vi "FIFORawDataScreener.vi"(2 "File Type":T2(ring)=enum."48 bit", 3 "Path":path) -> ()   [LabVIEW 2009]
uses:
  <vilib>/Analysis/NI_AALPro.lvlib
  <vilib>/Analysis/NI_AALBase.lvlib
panel:
  out "XY Graph":T1(graph)
  out "Waveform Graph":u32[](graph)
  out "MTOV B&H":dbl
  out "INV B&H":dbl
  out "MTOV & INV B&H":dbl
  out "MTOV & INV LV":dbl
  out "INV LV":dbl
  out "MTOV LV":dbl
  out "Waveform Graph 2":i32[](graph)
  in  "Bin":bool
  in  "proof":bool
  in  "Start":bool
  out "RawData":string[][](table)
  in  "Exit":bool
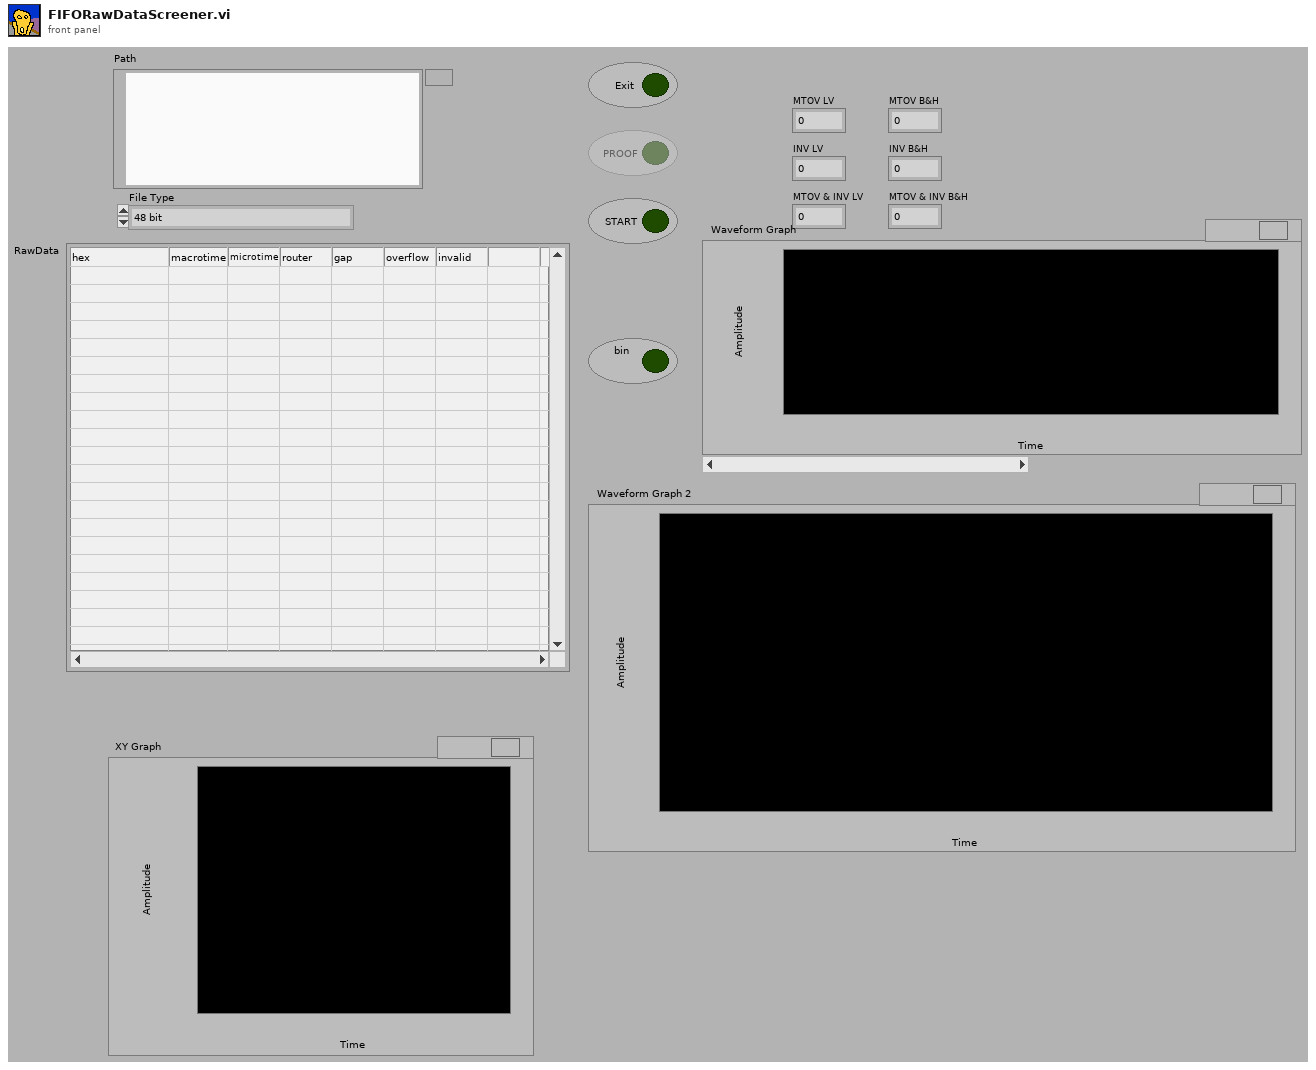
[diagram p1: front panel]
types:
  T1 = cluster{"X Values":dbl[], "Histogram: h(x)":i32[]}
  T2 = enum16{"32 bit", "48 bit", "48 bit (swapped bytes)", "32bit SPC830/130 LV Style", "32bit SPC830/130 B&H Style"}
  T3 = cluster{"router channels":u8[], "macro times":u32[], "micro times":u16[], "invalid times":u32[], "gap times":u32[]}
  T4 = enum16{"open", "open or create", "create or replace", "create", "open (read only)"}
  T5 = enum16{"Left Button", "Center Button", "Right Button", "Window Close"}
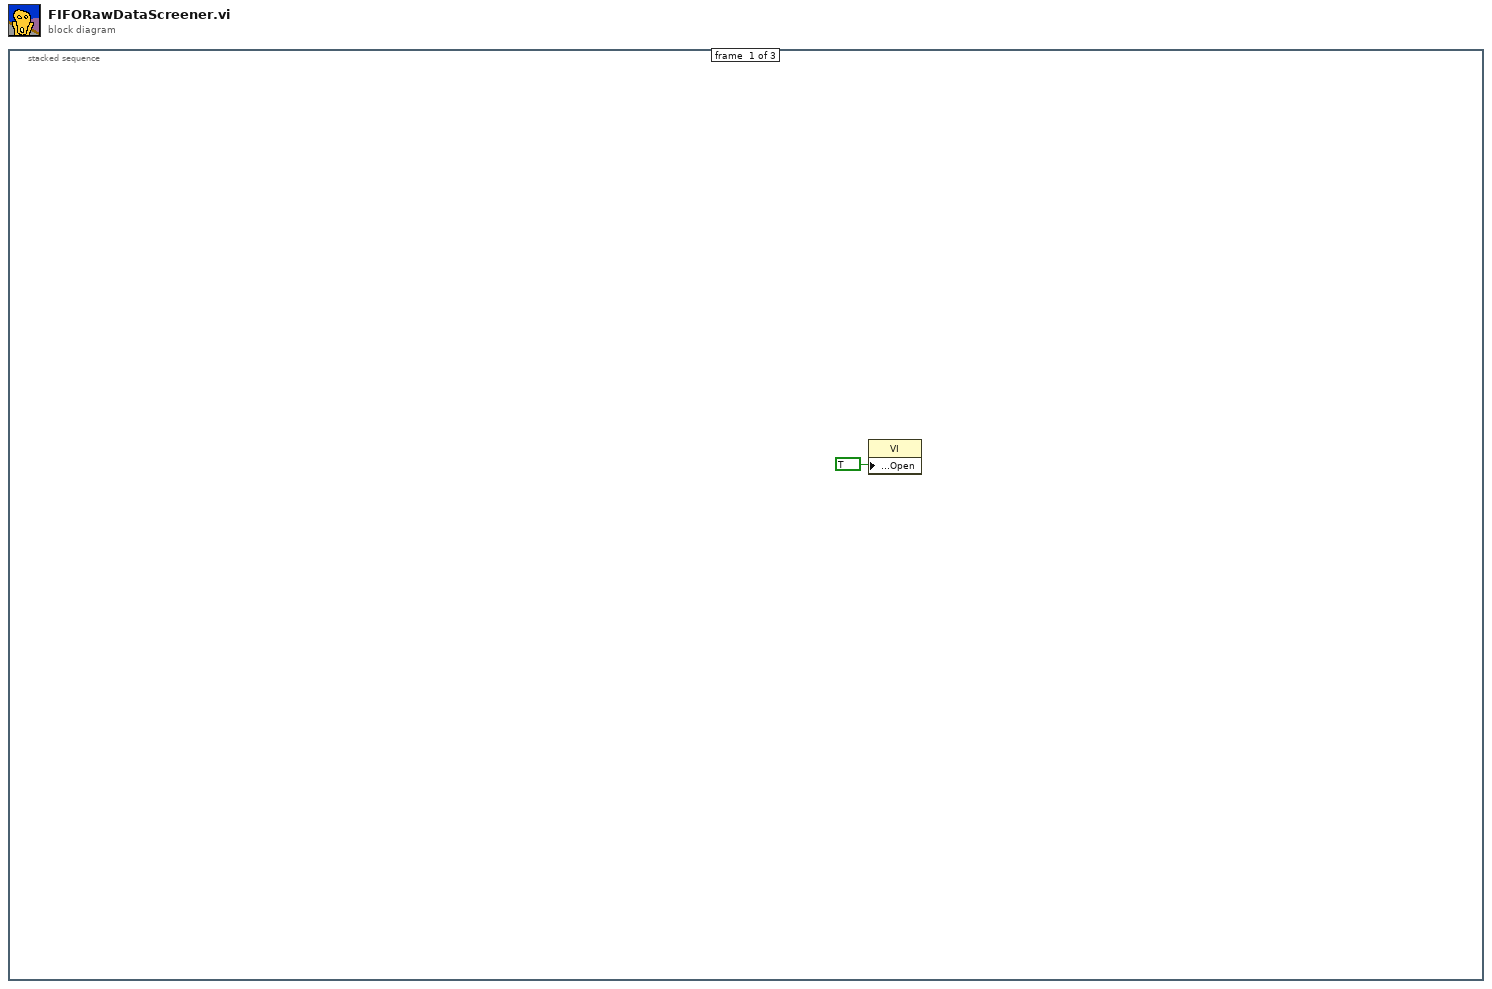
[diagram p0: block diagram]
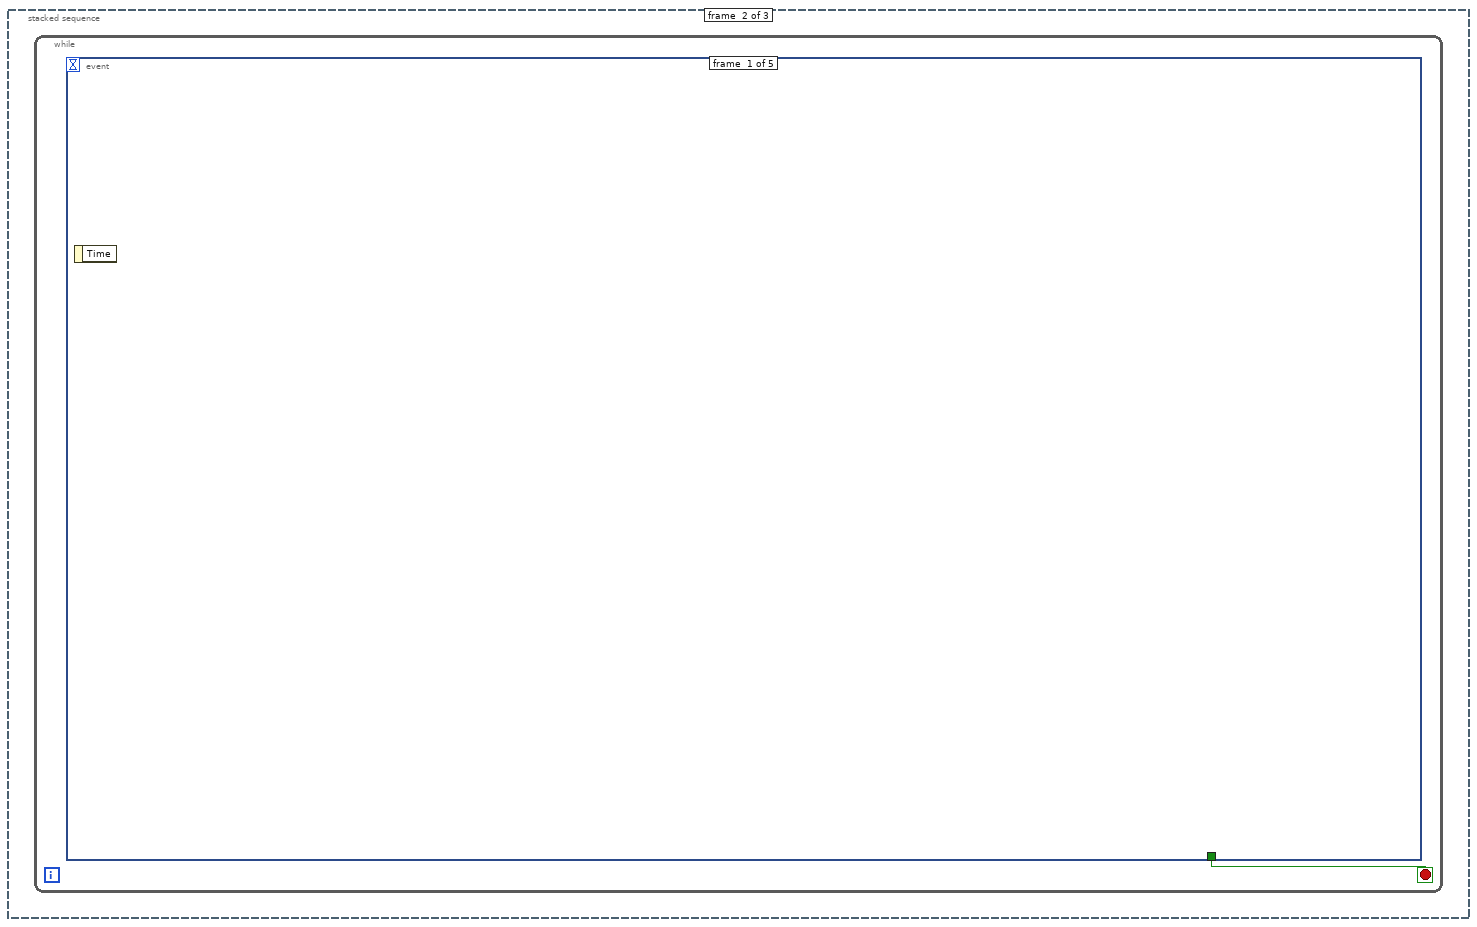
[diagram p2: hidden frame]
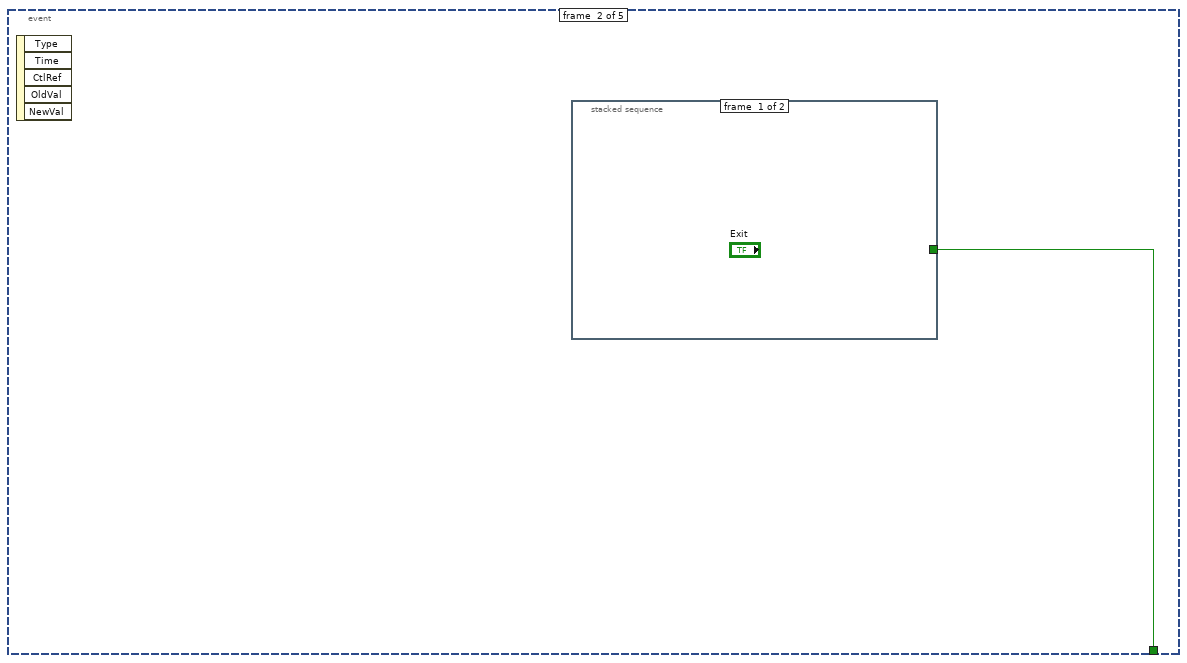
[diagram p3: hidden frame]
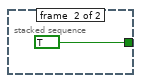
[diagram p4: hidden frame]
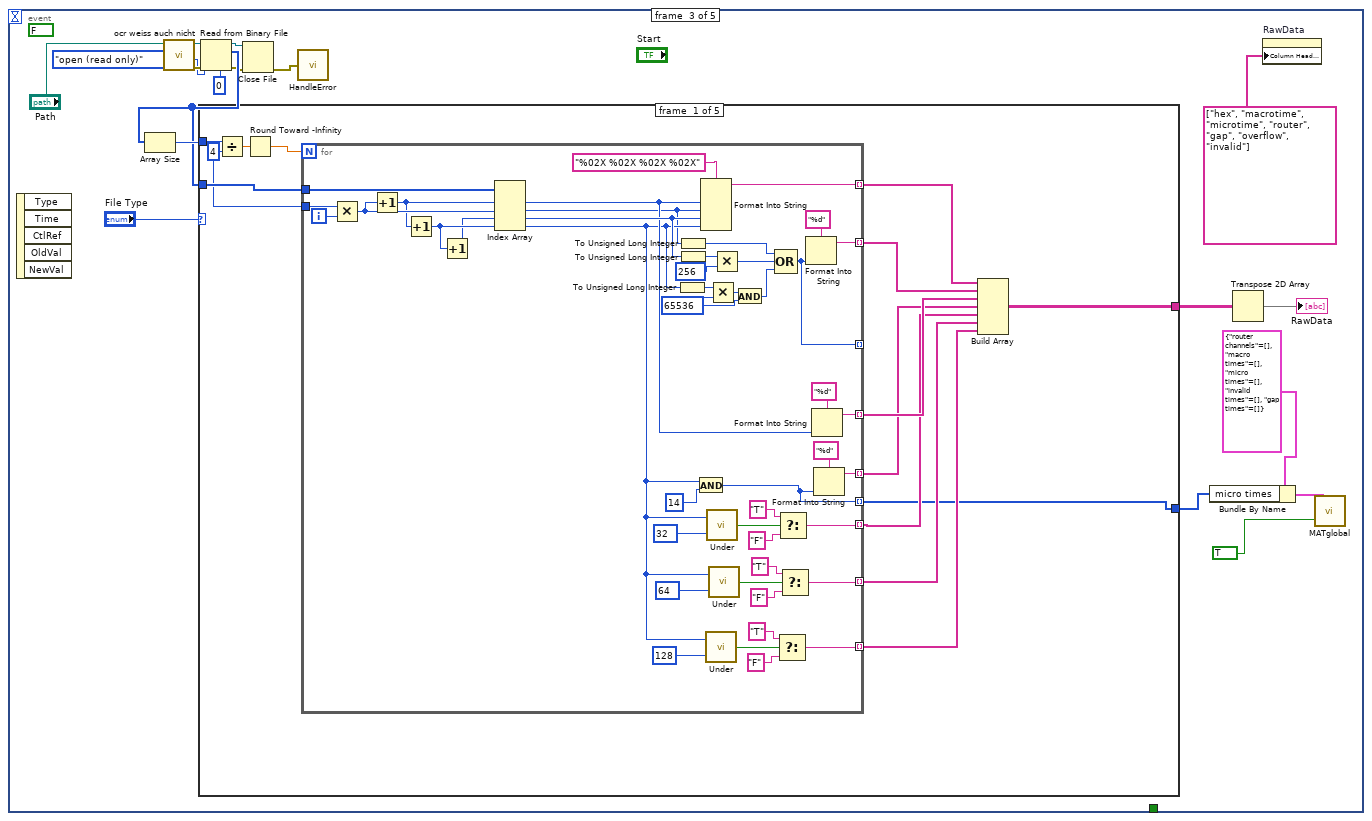
[diagram p5: hidden frame]
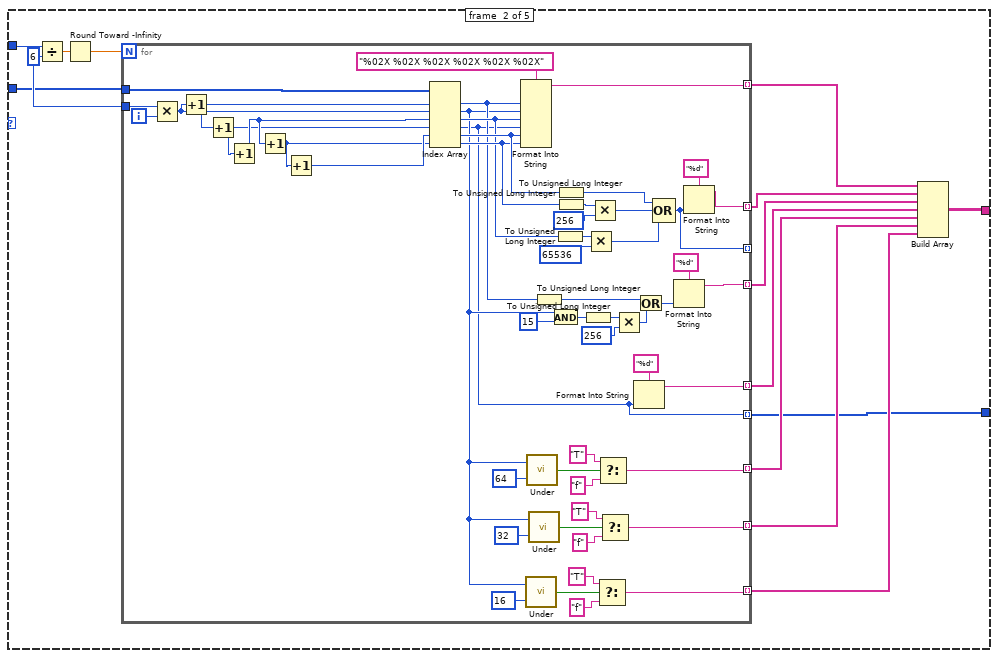
[diagram p6: hidden frame]
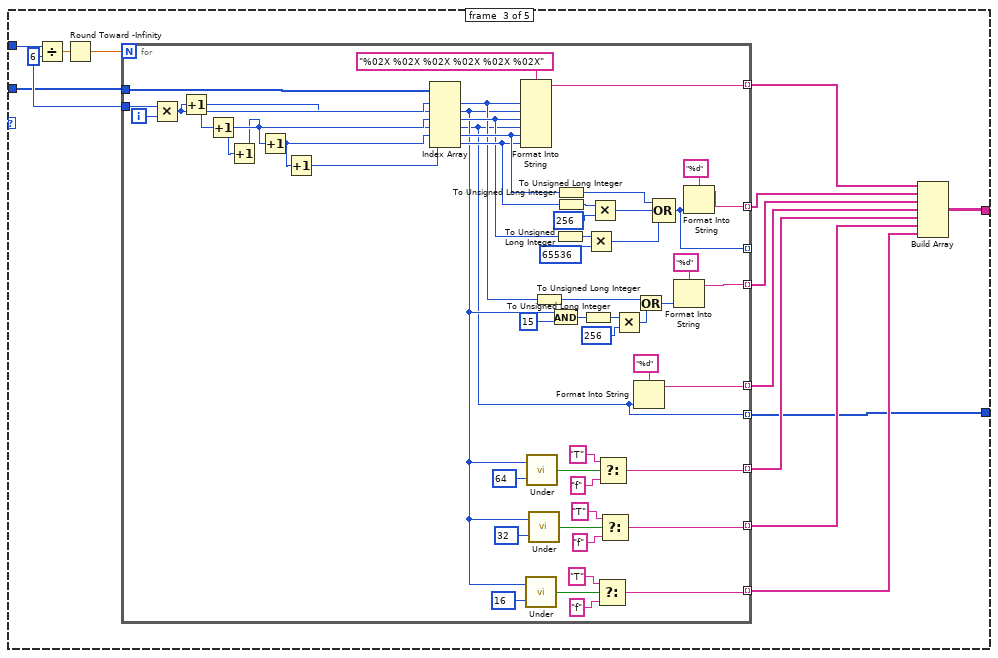
[diagram p7: hidden frame]
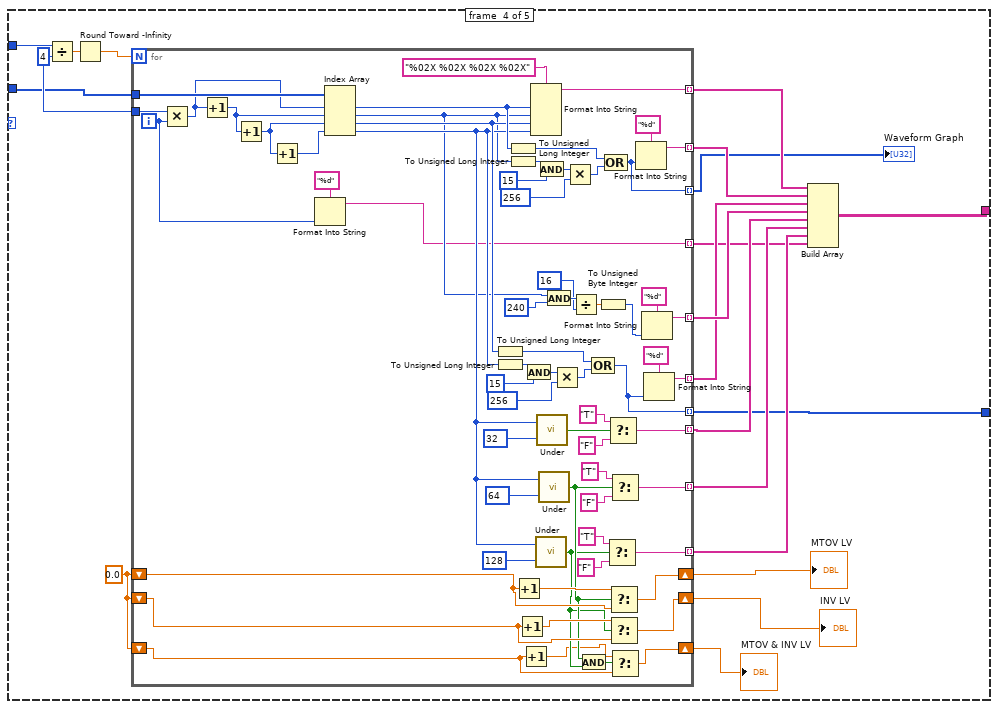
[diagram p8: hidden frame]
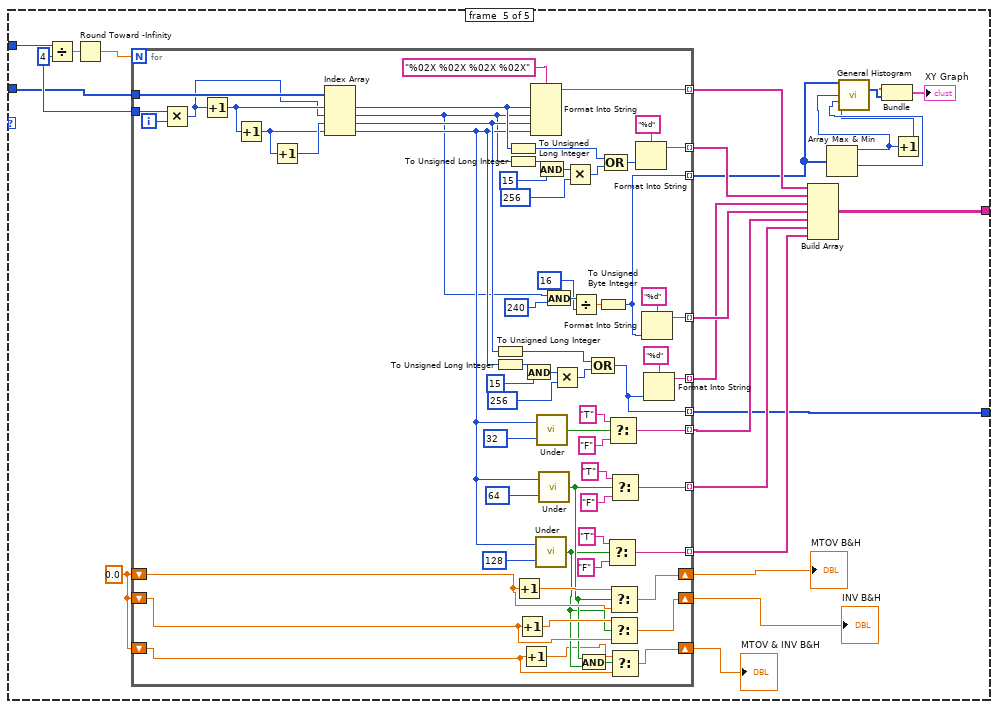
[diagram p9: hidden frame]
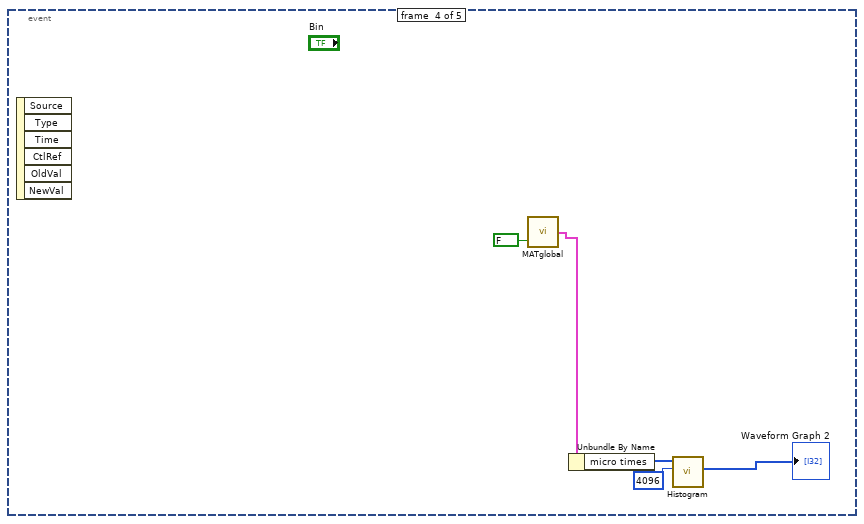
[diagram p10: hidden frame]
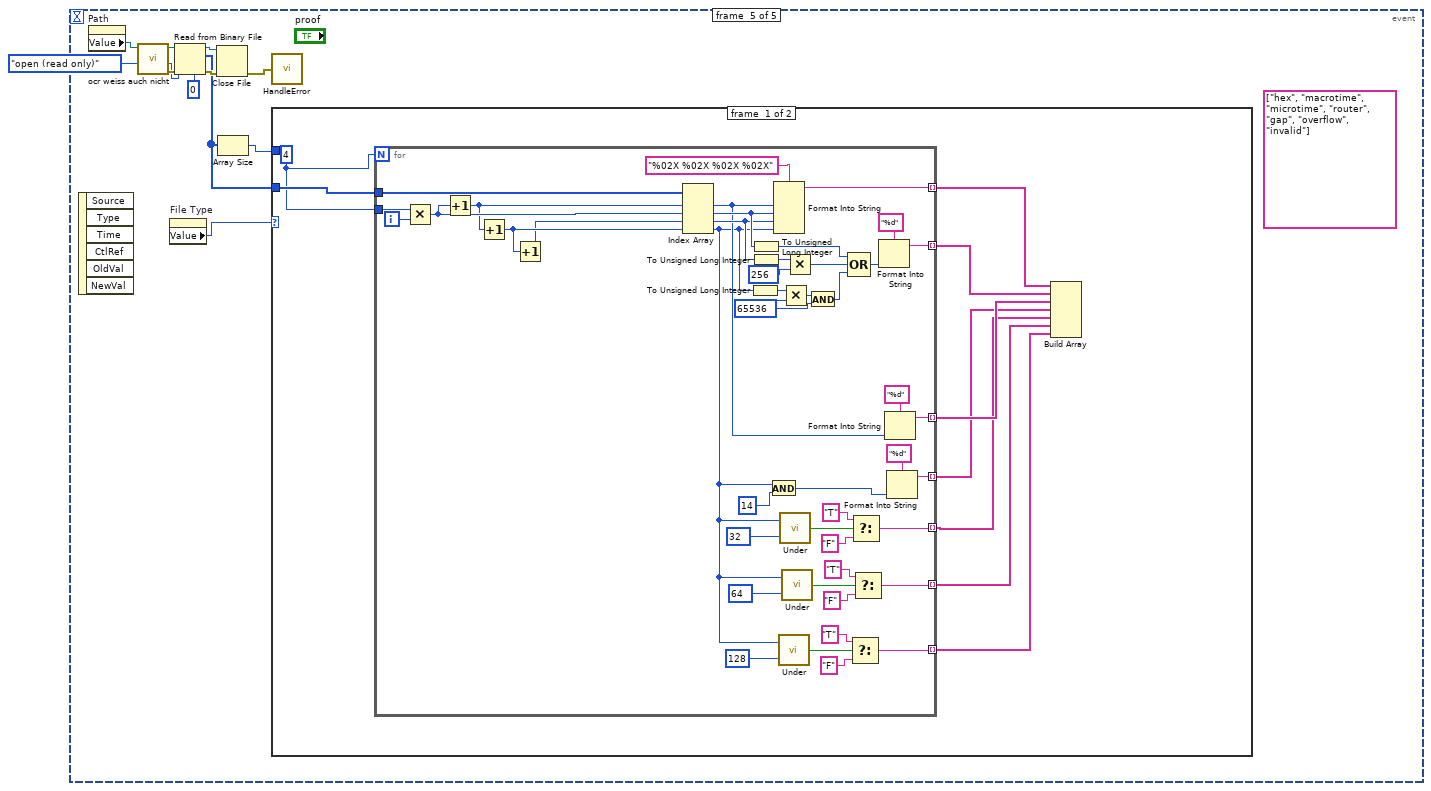
[diagram p11: hidden frame]
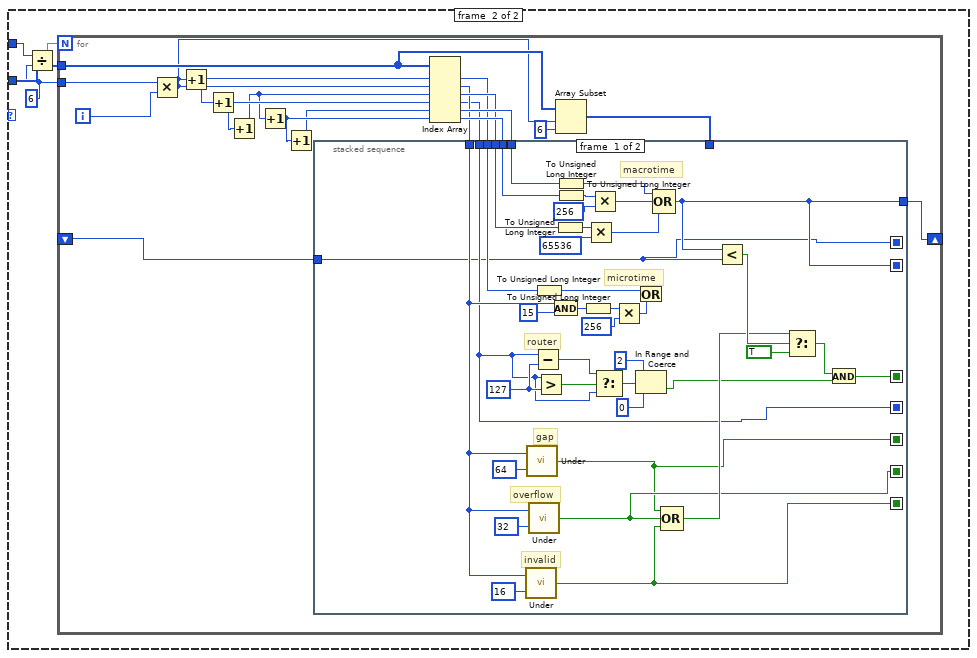
[diagram p12: hidden frame]
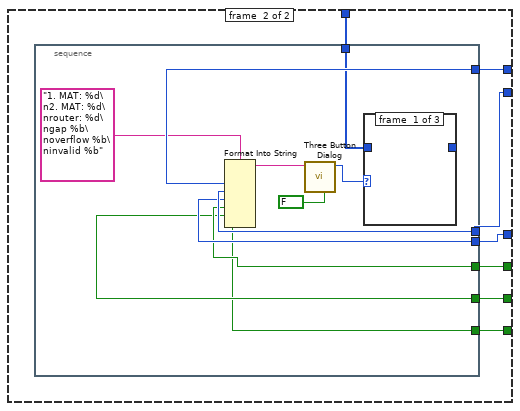
[diagram p14: hidden frame]
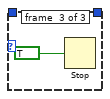
[diagram p16: hidden frame]
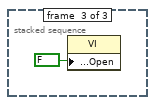
[diagram p17: hidden frame]
diagram:
  n1 = stacked-sequence {
    frame #0 {
      n2 = property class="VI"("Front Panel Window:Open"=TRUE) -> ()  [unwired: 2 in, 2 out]
    }
    frame #1 {
      n3 = while {
        stop <- w2 stop-if-true
        n4 = event shown="[2] \"Path\", \"File Type\", \"Start\": Value Change" {
          selector: _ -> [_ _ _ _ _]
          dyn-events: _ -> [_ _ _ _ _]
          timeout: _ -> [_ _ _ _ _]
          tunnel: [_ w3 _ _ _] -> w2
          event #0 {
            n5 = event-data() -> ()  [unwired: 1 in, 1 out]
          }
          event #1 {
            n6 = event-data() -> ()  [unwired: 1 in, 5 out]
            n7 = stacked-sequence {
              tunnel: [_ TRUE] -> w3
              frame #0 {
              }
              frame #1 {
              }
            }
          }
          event #2 {
            (unwired) FALSE
            n8 = event-data() -> ()  [unwired: 1 in, 5 out]
            n9 = call "ocr weiss auch nicht.vi"("function (open:0)"=T4."open (read only)", "file path"="Path") -> ("error out"=w15:errorcluster, "file size (bytes)"=w11:i32, "refnum"=w16:refnum<file>)  [unwired: 6 in, 1 out]
            n10 = Read from Binary File(5:u8 0 ("byte stream type"), 8:w15, 10:w11, 11:w16) -> (0:w12:errorcluster, 2:w21:u8[], 3:w13:refnum<file>)  [unwired: 2 in, 1 out]
            n11 = Array Size(array=w21) -> (size(s)=w22:i32)
            n12 = case shown="\"32bit SPC830/130 B&H Style\"" "File Type" {
              tunnel: w22 -> [w37 w86 w153 w227 w317]
              tunnel: w21 -> [w35 w83 w150 w228 w318]
              tunnel: [w25 w85 w152 w226 w316] -> w20
              tunnel: [w24 w84 w151 w223 w313] -> w5
              frame #0 {
                w34 = 4 ("y")
                n13 = Divide(x=w37, y=w34) -> (x/y=w36:dbl)
                n14 = Round Toward -Infinity(1:w36) -> (0:w33:dbl)
                n15 = for {
                  N: w33 -> [_]
                  tunnel: w35 -> [w82]
                  tunnel: w34 -> [w80]
                  tunnel: [w79] -> w32 mode=indexing
                  tunnel: [w68] -> w31 mode=indexing
                  tunnel: [w65] -> w30 mode=indexing
                  tunnel: [w63] -> w29 mode=indexing
                  tunnel: [w58] -> w28 mode=indexing
                  tunnel: [w49] -> w27 mode=indexing
                  tunnel: [w48] -> w26 mode=indexing
                  tunnel: [w39] -> _ mode=indexing
                  tunnel: [w38] -> w24 mode=indexing
                  i -> [w81]
                  w73 = u32 65536 ("y")
                  n16 = Multiply(x=w80, y=w81) -> (x*y=w44:i32)
                  n17 = Increment(x=w44) -> (x+1=w43:i32)
                  n18 = Increment(x=w43) -> (x+1=w42:i32)
                  n19 = Increment(x=w42) -> (x+1=w41:i32)
                  n20 = Index Array(array=w82, index #1=w43, index #2=w44, index #3=w41, index #4=w42) -> (element #1=w66:u8, element #2=w40:u8, element #3=w78:u8, element #4=w46:u8)
                  n21 = To Unsigned Long Integer(number=w46) -> (unsigned 32bit integer=w75:u32)
                  n22 = To Unsigned Long Integer(number=w40) -> (unsigned 32bit integer=w72:u32)
                  n23 = To Unsigned Long Integer(number=w78) -> (unsigned 32bit integer=w77:u32)
                  n24 = And(x=w46, y=u8 14) -> (x .and. y?=w38:u8)
                  n25 = Format Into String(format string="%02X %02X %02X %02X", w66, w40, w78, w46) -> (resulting string=w79:string)  [unwired: 2 in, 1 out]
                  n26 = call "Under.vi"("y"=u8 128, "byte stream type"=w46) -> ("Boolean"=w52:bool)
                  n27 = call "Under.vi"("y"=u8 32, "byte stream type"=w46) -> ("Boolean"=w61:bool)
                  n28 = Multiply(x=w75, y=w73) -> (x*y=w74:u32)
                  n29 = call "Under.vi"("y"=u8 64, "byte stream type"=w46) -> ("Boolean"=w55:bool)
                  n30 = Multiply(x=w77, y=u32 256) -> (x*y=w71:u32)
                  n31 = And(x=w74, y=w73) -> (x .and. y?=w70:u32)
                  n32 = Compound Arithmetic op=OR(w72, w71, w70) -> (w39:u32)
                  n33 = Select(t="T" ("format string"), s=w52, f="F" ("format string")) -> (s? t:f=w48:string)
                  n34 = Select(t="T" ("format string"), s=w61, f="F" ("format string")) -> (s? t:f=w58:string)
                  n35 = Select(t="T" ("format string"), s=w55, f="F" ("format string")) -> (s? t:f=w49:string)
                  n36 = Format Into String(format string="%d", w39) -> (resulting string=w68:string)  [unwired: 2 in, 1 out]
                  n37 = Format Into String(format string="%d", w66) -> (resulting string=w65:string)  [unwired: 2 in, 1 out]
                  n38 = Format Into String(format string="%d", w38) -> (resulting string=w63:string)  [unwired: 2 in, 1 out]
                }
                n39 = Build Array(w32, w31, w30, w29, w28, w27, w26) -> (w25:string[][])
              }
              frame #1 {
                w88 = 6 ("y")
                n40 = Divide(x=w86, y=w88) -> (x/y=w87:dbl)
                n41 = Round Toward -Infinity(1:w87) -> (0:w89:dbl)
                n42 = for {
                  N: w89 -> [_]
                  tunnel: w83 -> [w149]
                  tunnel: w88 -> [w147]
                  tunnel: [w145] -> w90 mode=indexing
                  tunnel: [w138] -> w91 mode=indexing
                  tunnel: [w136] -> w92 mode=indexing
                  tunnel: [w134] -> w93 mode=indexing
                  tunnel: [w129] -> w94 mode=indexing
                  tunnel: [w120] -> w95 mode=indexing
                  tunnel: [w119] -> w96 mode=indexing
                  tunnel: [w104] -> _ mode=indexing
                  tunnel: [w103] -> w84 mode=indexing
                  i -> [w148]
                  n43 = Multiply(x=w147, y=w148) -> (x*y=w101:i32)
                  n44 = Increment(x=w101) -> (x+1=w102:i32)
                  n45 = Increment(x=w102) -> (x+1=w99:i32)
                  n46 = Increment(x=w99) -> (x+1=w100:i32)
                  n47 = Increment(x=w100) -> (x+1=w97:i32)
                  n48 = Increment(x=w97) -> (x+1=w98:i32)
                  n49 = Index Array(array=w149, index #1=w102, index #2=w101, index #3=w100, index #4=w99, index #5=w98, index #6=w97) -> (element #1=w114:u8, element #2=w105:u8, element #3=w115:u8, element #4=w103:u8, element #5=w117:u8, element #6=w116:u8)
                  n50 = Format Into String(format string="%02X %02X %02X %02X %02X %02X", w114, w105, w115, w103, w117, w116) -> (resulting string=w145:string)  [unwired: 2 in, 1 out]
                  n51 = call "Under.vi"("y"=u8 16, "byte stream type"=w105) -> ("Boolean"=w123:bool)
                  n52 = call "Under.vi"("y"=u8 64, "byte stream type"=w105) -> ("Boolean"=w132:bool)
                  n53 = call "Under.vi"("y"=u8 32, "byte stream type"=w105) -> ("Boolean"=w126:bool)
                  n54 = To Unsigned Long Integer(number=w114) -> (unsigned 32bit integer=w109:u32)
                  n55 = And(x=w105, y=u8 15) -> (x .and. y?=w107:u8)
                  n56 = To Unsigned Long Integer(number=w115) -> (unsigned 32bit integer=w142:u32)
                  n57 = To Unsigned Long Integer(number=w117) -> (unsigned 32bit integer=w141:u32)
                  n58 = To Unsigned Long Integer(number=w116) -> (unsigned 32bit integer=w144:u32)
                  n59 = To Unsigned Long Integer(number=w107) -> (unsigned 32bit integer=w111:u32)
                  n60 = Multiply(x=w142, y=u32 65536) -> (x*y=w110:u32)
                  n61 = Multiply(x=w144, y=u32 256) -> (x*y=w140:u32)
                  n62 = Select(t="T" ("format string"), s=w123, f="f" ("format string")) -> (s? t:f=w119:string)
                  n63 = Select(t="T" ("format string"), s=w132, f="f" ("format string")) -> (s? t:f=w129:string)
                  n64 = Select(t="T" ("format string"), s=w126, f="f" ("format string")) -> (s? t:f=w120:string)
                  n65 = Multiply(x=w111, y=u32 256) -> (x*y=w108:u32)
                  n66 = Format Into String(format string="%d", w103) -> (resulting string=w134:string)  [unwired: 2 in, 1 out]
                  n67 = Or(x=w109, y=w108) -> (x .or. y?=w113:u32)
                  n68 = Compound Arithmetic op=OR(w141, w140, w110) -> (w104:u32)
                  n69 = Format Into String(format string="%d", w113) -> (resulting string=w136:string)  [unwired: 2 in, 1 out]
                  n70 = Format Into String(format string="%d", w104) -> (resulting string=w138:string)  [unwired: 2 in, 1 out]
                }
                n71 = Build Array(w90, w91, w92, w93, w94, w95, w96) -> (w85:string[][])
              }
              frame #2 {
                w155 = 6 ("y")
                n72 = Divide(x=w153, y=w155) -> (x/y=w154:dbl)
                n73 = Round Toward -Infinity(1:w154) -> (0:w156:dbl)
                n74 = for {
                  N: w156 -> [_]
                  tunnel: w150 -> [w216]
                  tunnel: w155 -> [w214]
                  tunnel: [w212] -> w157 mode=indexing
                  tunnel: [w205] -> w158 mode=indexing
                  tunnel: [w203] -> w159 mode=indexing
                  tunnel: [w201] -> w160 mode=indexing
                  tunnel: [w196] -> w161 mode=indexing
                  tunnel: [w187] -> w162 mode=indexing
                  tunnel: [w186] -> w163 mode=indexing
                  tunnel: [w171] -> _ mode=indexing
                  tunnel: [w170] -> w151 mode=indexing
                  i -> [w215]
                  n75 = Multiply(x=w214, y=w215) -> (x*y=w169:i32)
                  n76 = Increment(x=w169) -> (x+1=w168:i32)
                  n77 = Increment(x=w168) -> (x+1=w167:i32)
                  n78 = Increment(x=w167) -> (x+1=w166:i32)
                  n79 = Increment(x=w166) -> (x+1=w165:i32)
                  n80 = Increment(x=w165) -> (x+1=w164:i32)
                  n81 = Index Array(array=w216, index #1=w169, index #2=w168, index #3=w167, index #4=w166, index #5=w165, index #6=w164) -> (element #1=w181:u8, element #2=w172:u8, element #3=w182:u8, element #4=w170:u8, element #5=w184:u8, element #6=w183:u8)
                  n82 = Format Into String(format string="%02X %02X %02X %02X %02X %02X", w181, w172, w182, w170, w184, w183) -> (resulting string=w212:string)  [unwired: 2 in, 1 out]
                  n83 = call "Under.vi"("y"=u8 16, "byte stream type"=w172) -> ("Boolean"=w190:bool)
                  n84 = call "Under.vi"("y"=u8 64, "byte stream type"=w172) -> ("Boolean"=w199:bool)
                  n85 = call "Under.vi"("y"=u8 32, "byte stream type"=w172) -> ("Boolean"=w193:bool)
                  n86 = To Unsigned Long Integer(number=w181) -> (unsigned 32bit integer=w176:u32)
                  n87 = And(x=w172, y=u8 15) -> (x .and. y?=w174:u8)
                  n88 = To Unsigned Long Integer(number=w182) -> (unsigned 32bit integer=w209:u32)
                  n89 = To Unsigned Long Integer(number=w184) -> (unsigned 32bit integer=w208:u32)
                  n90 = To Unsigned Long Integer(number=w183) -> (unsigned 32bit integer=w211:u32)
                  n91 = To Unsigned Long Integer(number=w174) -> (unsigned 32bit integer=w178:u32)
                  n92 = Multiply(x=w209, y=u32 65536) -> (x*y=w177:u32)
                  n93 = Multiply(x=w211, y=u32 256) -> (x*y=w207:u32)
                  n94 = Select(t="T" ("format string"), s=w190, f="f" ("format string")) -> (s? t:f=w186:string)
                  n95 = Select(t="T" ("format string"), s=w199, f="f" ("format string")) -> (s? t:f=w196:string)
                  n96 = Select(t="T" ("format string"), s=w193, f="f" ("format string")) -> (s? t:f=w187:string)
                  n97 = Multiply(x=w178, y=u32 256) -> (x*y=w175:u32)
                  n98 = Format Into String(format string="%d", w170) -> (resulting string=w201:string)  [unwired: 2 in, 1 out]
                  n99 = Or(x=w176, y=w175) -> (x .or. y?=w180:u32)
                  n100 = Compound Arithmetic op=OR(w208, w207, w177) -> (w171:u32)
                  n101 = Format Into String(format string="%d", w180) -> (resulting string=w203:string)  [unwired: 2 in, 1 out]
                  n102 = Format Into String(format string="%d", w171) -> (resulting string=w205:string)  [unwired: 2 in, 1 out]
                }
                n103 = Build Array(w157, w158, w159, w160, w161, w162, w163) -> (w152:string[][])
              }
              frame #3 {
                w220 = 0.0
                w235 = 4 ("y")
                n104 = Divide(x=w227, y=w235) -> (x/y=w236:dbl)
                n105 = Round Toward -Infinity(1:w236) -> (0:w234:dbl)
                n106 = for {
                  N: w234 -> [_]
                  tunnel: w228 -> [w301]
                  tunnel: w235 -> [w300]
                  tunnel: [w299] -> w233 mode=indexing
                  tunnel: [w296] -> w232 mode=indexing
                  tunnel: [w294] -> w225 mode=indexing
                  tunnel: [w292] -> w224 mode=indexing
                  tunnel: [w287] -> w231 mode=indexing
                  tunnel: [w281] -> w230 mode=indexing
                  tunnel: [w280] -> w229 mode=indexing
                  tunnel: [w241] -> w223 mode=indexing
                  shift-right: [w249] -> w222
                  shift-left: w220 -> [w250]
                  shift-right: [w254] -> w221
                  shift-left: w220 -> [w253]
                  shift-right: [w248] -> w219
                  shift-left: w220 -> [w243]
                  tunnel: [w240] -> w218 mode=indexing
                  tunnel: [w237] -> w217 mode=indexing
                  i -> [w238]
                  n107 = Multiply(x=w300, y=w238) -> (x*y=w259:i32)
                  n108 = Increment(x=w259) -> (x+1=w258:i32)
                  n109 = Increment(x=w258) -> (x+1=w257:i32)
                  n110 = Increment(x=w257) -> (x+1=w256:i32)
                  n111 = Format Into String(format string="%d", w238) -> (resulting string=w237:string)  [unwired: 2 in, 1 out]
                  n112 = Index Array(array=w301, index #1=w259, index #2=w258, index #3=w257, index #4=w256) -> (element #1=w278:u8, element #2=w263:u8, element #3=w266:u8, element #4=w265:u8)
                  n113 = To Unsigned Long Integer(number=w266) -> (unsigned 32bit integer=w267:u32)
                  n114 = To Unsigned Long Integer(number=w265) -> (unsigned 32bit integer=w269:u32)
                  n115 = To Unsigned Long Integer(number=w278) -> (unsigned 32bit integer=w298:u32)
                  n116 = To Unsigned Long Integer(number=w263) -> (unsigned 32bit integer=w276:u32)
                  n117 = Increment(x=w250) -> (x+1=w251:dbl)
                  n118 = Increment(x=w253) -> (x+1=w252:dbl)
                  n119 = Increment(x=w243) -> (x+1=w244:dbl)
                  n120 = And(x=w269, y=u32 15) -> (x .and. y?=w270:u32)
                  n121 = Format Into String(format string="%02X %02X %02X %02X", w278, w263, w266, w265) -> (resulting string=w299:string)  [unwired: 2 in, 1 out]
                  n122 = call "Under.vi"("y"=u8 128, "byte stream type"=w265) -> ("Boolean"=w245:bool)
                  n123 = And(x=w276, y=u32 15) -> (x .and. y?=w275:u32)
                  n124 = call "Under.vi"("y"=u8 32, "byte stream type"=w265) -> ("Boolean"=w290:bool)
                  n125 = call "Under.vi"("y"=u8 64, "byte stream type"=w265) -> ("Boolean"=w246:bool)
                  n126 = And(x=w263, y=u8 240) -> (x .and. y?=w262:u8)
                  n127 = Multiply(x=w270, y=u32 256) -> (x*y=w272:u32)
                  n128 = Multiply(x=w275, y=u32 256) -> (x*y=w273:u32)
                  n129 = Divide(x=w262, y=u8 16) -> (x/y=w260:dbl)
                  n130 = And(x=w246, y=w245) -> (x .and. y?=w247:bool)
                  n131 = Compound Arithmetic op=OR(w267, w272) -> (w241:u32)
                  n132 = To Unsigned Byte Integer(number=w260) -> (unsigned 8bit integer=w242:u8)
                  n133 = Compound Arithmetic op=OR(w298, w273) -> (w240:u32)
                  n134 = Select(t="T" ("format string"), s=w245, f="F" ("format string")) -> (s? t:f=w280:string)
                  n135 = Select(t="T" ("format string"), s=w290, f="F" ("format string")) -> (s? t:f=w287:string)
                  n136 = Select(t=w251, s=w246, f=w250) -> (s? t:f=w249:dbl)
                  n137 = Select(t=w252, s=w245, f=w253) -> (s? t:f=w254:dbl)
                  n138 = Select(t="T" ("format string"), s=w246, f="F" ("format string")) -> (s? t:f=w281:string)
                  n139 = Select(t=w244, s=w247, f=w243) -> (s? t:f=w248:dbl)
                  n140 = Format Into String(format string="%d", w240) -> (resulting string=w296:string)  [unwired: 2 in, 1 out]
                  n141 = Format Into String(format string="%d", w242) -> (resulting string=w294:string)  [unwired: 2 in, 1 out]
                  n142 = Format Into String(format string="%d", w241) -> (resulting string=w292:string)  [unwired: 2 in, 1 out]
                }
                "MTOV LV" <- w222
                "INV LV" <- w221
                "MTOV & INV LV" <- w219
                "Waveform Graph" <- w218
                n143 = Build Array(w233, w232, w224, w225, w231, w230, w229, w217) -> (w226:string[][])
              }
              frame #4 {
                w310 = 0.0
                w325 = 4 ("y")
                n144 = Divide(x=w317, y=w325) -> (x/y=w326:dbl)
                n145 = Round Toward -Infinity(1:w326) -> (0:w324:dbl)
                n146 = for {
                  N: w324 -> [_]
                  tunnel: w318 -> [w389]
                  tunnel: w325 -> [w387]
                  tunnel: [w386] -> w323 mode=indexing
                  tunnel: [w383] -> w322 mode=indexing
                  tunnel: [w381] -> w315 mode=indexing
                  tunnel: [w379] -> w314 mode=indexing
                  tunnel: [w374] -> w321 mode=indexing
                  tunnel: [w368] -> w320 mode=indexing
                  tunnel: [w367] -> w319 mode=indexing
                  tunnel: [w345] -> w313 mode=indexing
                  shift-right: [w338] -> w312
                  shift-left: w310 -> [w339]
                  shift-right: [w343] -> w311
                  shift-left: w310 -> [w342]
                  shift-right: [w337] -> w309
                  shift-left: w310 -> [w332]
                  tunnel: [w327] -> w305 mode=indexing
                  i -> [w388]
                  n147 = Multiply(x=w387, y=w388) -> (x*y=w330:i32)
                  n148 = Increment(x=w330) -> (x+1=w331:i32)
                  n149 = Increment(x=w331) -> (x+1=w328:i32)
                  n150 = Increment(x=w328) -> (x+1=w329:i32)
                  n151 = Index Array(array=w389, index #1=w331, index #2=w330, index #3=w329, index #4=w328) -> (element #1=w365:u8, element #2=w350:u8, element #3=w353:u8, element #4=w352:u8)
                  n152 = To Unsigned Long Integer(number=w353) -> (unsigned 32bit integer=w354:u32)
                  n153 = To Unsigned Long Integer(number=w352) -> (unsigned 32bit integer=w356:u32)
                  n154 = To Unsigned Long Integer(number=w365) -> (unsigned 32bit integer=w385:u32)
                  n155 = To Unsigned Long Integer(number=w350) -> (unsigned 32bit integer=w363:u32)
                  n156 = Increment(x=w339) -> (x+1=w340:dbl)
                  n157 = Increment(x=w342) -> (x+1=w341:dbl)
                  n158 = Increment(x=w332) -> (x+1=w333:dbl)
                  n159 = And(x=w356, y=u32 15) -> (x .and. y?=w357:u32)
                  n160 = Format Into String(format string="%02X %02X %02X %02X", w365, w350, w353, w352) -> (resulting string=w386:string)  [unwired: 2 in, 1 out]
                  n161 = call "Under.vi"("y"=u8 128, "byte stream type"=w352) -> ("Boolean"=w334:bool)
                  n162 = And(x=w363, y=u32 15) -> (x .and. y?=w362:u32)
                  n163 = call "Under.vi"("y"=u8 32, "byte stream type"=w352) -> ("Boolean"=w377:bool)
                  n164 = call "Under.vi"("y"=u8 64, "byte stream type"=w352) -> ("Boolean"=w335:bool)
                  n165 = And(x=w350, y=u8 240) -> (x .and. y?=w349:u8)
                  n166 = Multiply(x=w357, y=u32 256) -> (x*y=w359:u32)
                  n167 = Multiply(x=w362, y=u32 256) -> (x*y=w360:u32)
                  n168 = Divide(x=w349, y=u8 16) -> (x/y=w347:dbl)
                  n169 = And(x=w335, y=w334) -> (x .and. y?=w336:bool)
                  n170 = Compound Arithmetic op=OR(w354, w359) -> (w345:u32)
                  n171 = To Unsigned Byte Integer(number=w347) -> (unsigned 8bit integer=w327:u8)
                  n172 = Compound Arithmetic op=OR(w385, w360) -> (w346:u32)
                  n173 = Select(t="T" ("format string"), s=w334, f="F" ("format string")) -> (s? t:f=w367:string)
                  n174 = Select(t="T" ("format string"), s=w377, f="F" ("format string")) -> (s? t:f=w374:string)
                  n175 = Select(t=w340, s=w335, f=w339) -> (s? t:f=w338:dbl)
                  n176 = Select(t=w341, s=w334, f=w342) -> (s? t:f=w343:dbl)
                  n177 = Select(t="T" ("format string"), s=w335, f="F" ("format string")) -> (s? t:f=w368:string)
                  n178 = Select(t=w333, s=w336, f=w332) -> (s? t:f=w337:dbl)
                  n179 = Format Into String(format string="%d", w346) -> (resulting string=w383:string)  [unwired: 2 in, 1 out]
                  n180 = Format Into String(format string="%d", w327) -> (resulting string=w381:string)  [unwired: 2 in, 1 out]
                  n181 = Format Into String(format string="%d", w345) -> (resulting string=w379:string)  [unwired: 2 in, 1 out]
                }
                "MTOV B&H" <- w312
                "INV B&H" <- w311
                "MTOV & INV B&H" <- w309
                n182 = Build Array(w323, w322, w314, w315, w321, w320, w319) -> (w316:string[][])
                n183 = Array Max & Min(array=w305) -> (max value=w303:u8, min value=w304:u8)  [unwired: 2 out]
                n184 = Increment(x=w303) -> (x+1=w302:u8)
                n185 = call <vilib>:"General Histogram.vi"("X"=w305, "max"=w303, "min"=w304, "# bins"=w302) -> ("Histogram"=w307:i32[], "Axis"=w306:dbl[])  [unwired: 7 in, 3 out]
                n186 = Bundle("Axis"=w306, "Histogram"=w307) -> (→"XY Graph":cluster{"Axis":dbl[], "Histogram":i32[]})  [unwired: 1 in]
              }
            }
            n187 = Close File(refnum=w13, error in=w12) -> (error out=w9:errorcluster)  [unwired: 1 out]
            n188 = call "HandleError.vi"("error in (no error)"=w9) -> ()
            n189 = Bundle By Name(cluster=T3 {"router channels"=[], "macro times"=[], "micro times"=[], "invalid times"=[], "gap times"=[]} ("rawdata"), "micro times"=w5) -> (w6:T3)
            n190 = Transpose 2D Array(2D array=w20) -> (transposed array=→"RawData":string[][])
            n191 = property on="RawData" class="Tbl (strict)"("Column Header Strings[]"=string[] ["hex", "macrotime", "microtime", "router", "gap", "overflow", "invalid"] ("Column Headers[]")) -> ()  [unwired: 2 in, 2 out]
            n192 = call "MATglobal.vi"("s"=TRUE, "rawdata"=w6) -> ()  [unwired: 1 out]
          }
          event #3 {
            n193 = event-data() -> ()  [unwired: 1 in, 6 out]
            n194 = call "MATglobal.vi"("s"=FALSE) -> ("rawdata"=w393:T3)  [unwired: 1 in]
            n195 = Unbundle By Name(w393) -> ("micro times"=w392:u16[])
            n196 = call <vilib>:"Histogram.vi"("intervals"=4096, "X"=w392) -> ("Histogram: h(x)"=→"Waveform Graph 2":i32[])  [unwired: 6 in, 3 out]
          }
          event #4 {
            (unwired) string[] ["hex", "macrotime", "microtime", "router", "gap", "overflow", "invalid"] ("Column Headers[]")
            n197 = event-data() -> ()  [unwired: 1 in, 6 out]
            n198 = property on="Path" class="Path"() -> ("Value"=w397:path)  [unwired: 2 in, 2 out]
            n199 = call "ocr weiss auch nicht.vi"("function (open:0)"=T4."open (read only)", "file path"=w397) -> ("error out"=w405:errorcluster, "file size (bytes)"=w401:i32, "refnum"=w406:refnum<file>)  [unwired: 6 in, 1 out]
            n200 = property on="File Type" class="Enum (strict)"() -> ("Value"=w396:T2)  [unwired: 2 in, 2 out]
            n201 = Read from Binary File(5:u8 0 ("byte stream type"), 8:w405, 10:w401, 11:w406) -> (0:w402:errorcluster, 2:w400:u8[], 3:w403:refnum<file>)  [unwired: 2 in, 1 out]
            n202 = Close File(refnum=w403, error in=w402) -> (error out=w398:errorcluster)  [unwired: 1 out]
            n203 = Array Size(array=w400) -> (size(s)=w395:i32)
            n204 = call "HandleError.vi"("error in (no error)"=w398) -> ()
            n205 = case shown="\"32 bit\", Default" w396 {
              tunnel: w400 -> [w415 w464]
              tunnel: w395 -> [_ w462]
              frame #0 {
                w407 = 4 ("y")
                n206 = for {
                  N: w407 -> [_]
                  tunnel: w415 -> [w460]
                  tunnel: w407 -> [w458]
                  tunnel: [w457] -> w414 mode=indexing
                  tunnel: [w444] -> w413 mode=indexing
                  tunnel: [w441] -> w412 mode=indexing
                  tunnel: [w439] -> w411 mode=indexing
                  tunnel: [w434] -> w410 mode=indexing
                  tunnel: [w425] -> w409 mode=indexing
                  tunnel: [w424] -> w408 mode=indexing
                  i -> [w459]
                  w450 = u32 65536 ("y")
                  n207 = Multiply(x=w458, y=w459) -> (x*y=w419:i32)
                  n208 = Increment(x=w419) -> (x+1=w418:i32)
                  n209 = Increment(x=w418) -> (x+1=w417:i32)
                  n210 = Increment(x=w417) -> (x+1=w416:i32)
                  n211 = Index Array(array=w460, index #1=w418, index #2=w419, index #3=w416, index #4=w417) -> (element #1=w442:u8, element #2=w456:u8, element #3=w455:u8, element #4=w422:u8)
                  n212 = To Unsigned Long Integer(number=w422) -> (unsigned 32bit integer=w452:u32)
                  n213 = To Unsigned Long Integer(number=w456) -> (unsigned 32bit integer=w449:u32)
                  n214 = To Unsigned Long Integer(number=w455) -> (unsigned 32bit integer=w454:u32)
                  n215 = And(x=w422, y=u8 14) -> (x .and. y?=w420:u8)
                  n216 = Format Into String(format string="%02X %02X %02X %02X", w442, w456, w455, w422) -> (resulting string=w457:string)  [unwired: 2 in, 1 out]
                  n217 = call "Under.vi"("y"=u8 128, "byte stream type"=w422) -> ("Boolean"=w428:bool)
                  n218 = call "Under.vi"("y"=u8 32, "byte stream type"=w422) -> ("Boolean"=w437:bool)
                  n219 = Multiply(x=w452, y=w450) -> (x*y=w451:u32)
                  n220 = call "Under.vi"("y"=u8 64, "byte stream type"=w422) -> ("Boolean"=w431:bool)
                  n221 = Multiply(x=w454, y=u32 256) -> (x*y=w448:u32)
                  n222 = And(x=w451, y=w450) -> (x .and. y?=w447:u32)
                  n223 = Compound Arithmetic op=OR(w449, w448, w447) -> (w445:u32)
                  n224 = Select(t="T" ("format string"), s=w428, f="F" ("format string")) -> (s? t:f=w424:string)
                  n225 = Select(t="T" ("format string"), s=w437, f="F" ("format string")) -> (s? t:f=w434:string)
                  n226 = Select(t="T" ("format string"), s=w431, f="F" ("format string")) -> (s? t:f=w425:string)
                  n227 = Format Into String(format string="%d", w445) -> (resulting string=w444:string)  [unwired: 2 in, 1 out]
                  n228 = Format Into String(format string="%d", w442) -> (resulting string=w441:string)  [unwired: 2 in, 1 out]
                  n229 = Format Into String(format string="%d", w420) -> (resulting string=w439:string)  [unwired: 2 in, 1 out]
                }
                n230 = Build Array(w414, w413, w412, w411, w410, w409, w408) -> ()  [unwired: 1 out]
              }
              frame #1 {
                w461 = 6 ("y")
                n231 = Divide(x=w462, y=w461) -> (x/y=w463:dbl)
                n232 = for {
                  N: w463 -> [_]
                  tunnel: w464 -> [w468]
                  tunnel: w461 -> [w482]
                  shift-right: [w481] -> _
                  shift-left: _ -> [w480]
                  i -> [w483]
                  n233 = Multiply(x=w482, y=w483) -> (x*y=w467:i32)
                  n234 = Increment(x=w467) -> (x+1=w474:i32)
                  n235 = Increment(x=w474) -> (x+1=w471:i32)
                  n236 = Increment(x=w471) -> (x+1=w470:i32)
                  n237 = Increment(x=w470) -> (x+1=w473:i32)
                  n238 = Increment(x=w473) -> (x+1=w472:i32)
                  n239 = Index Array(array=w468, index #1=w474, index #2=w467, index #3=w470, index #4=w471, index #5=w472, index #6=w473) -> (element #1=w476:u8, element #2=w475:u8, element #3=w477:u8, element #4=w469:u8, element #5=w479:u8, element #6=w478:u8)
                  n240 = Array Subset(array=w468, index=w467, length=6) -> (w465:u8[])
                  n241 = stacked-sequence {
                    seq-local: [w490 _] -> [_ w530]
                    seq-local: [w484 _] -> [_ w529]
                    seq-local: [w485 _] -> [_ w528]
                    seq-local: [w486 _] -> [_ w527]
                    seq-local: [w487 _] -> [_ w526]
                    seq-local: [w488 _] -> [_ w525]
                    seq-local: [w489 _] -> [_ w524]
                    tunnel: [w485 _] -> w481
                    tunnel: w480 -> [w484 _]
                    tunnel: w479 -> [w513 _]
                    tunnel: w478 -> [w512 _]
                    tunnel: w477 -> [w511 _]
                    tunnel: w476 -> [w510 _]
                    tunnel: w475 -> [w502 _]
                    tunnel: w469 -> [w486 _]
                    tunnel: w465 -> [_ w523]
                    frame #0 {
                      w496 = u8 127 ("y")
                      # "macrotime"
                      # "microtime"
                      # "router"
                      # "invalid"
                      # "overflow"
                      # "gap"
                      n242 = call "Under.vi"("y"=u8 16, "byte stream type"=w502) -> ("Boolean"=w489:bool)
                      n243 = call "Under.vi"("y"=u8 64, "byte stream type"=w502) -> ("Boolean"=w487:bool)
                      n244 = call "Under.vi"("y"=u8 32, "byte stream type"=w502) -> ("Boolean"=w488:bool)
                      n245 = Subtract(x=w486, y=w496) -> (x-y=w495:u8)
                      n246 = To Unsigned Long Integer(number=w510) -> (unsigned 32bit integer=w506:u32)
                      n247 = Greater?(x=w486, y=w496) -> (0:w497:bool)
                      n248 = And(x=w502, y=u8 15) -> (x .and. y?=w504:u8)
                      n249 = To Unsigned Long Integer(number=w511) -> (unsigned 32bit integer=w520:u32)
                      n250 = To Unsigned Long Integer(number=w513) -> (unsigned 32bit integer=w519:u32)
                      n251 = To Unsigned Long Integer(number=w512) -> (unsigned 32bit integer=w522:u32)
                      n252 = To Unsigned Long Integer(number=w504) -> (unsigned 32bit integer=w508:u32)
                      n253 = Multiply(x=w520, y=u32 65536) -> (x*y=w507:u32)
                      n254 = Multiply(x=w522, y=u32 256) -> (x*y=w518:u32)
                      n255 = Select(t=w495, s=w497, f=w486) -> (s? t:f=w494:u8)
                      n256 = Multiply(x=w508, y=u32 256) -> (x*y=w505:u32)
                      n257 = Or(x=w506, y=w505) -> ()  [unwired: 1 out]
                      n258 = In Range and Coerce(upper limit=u8 2, x=w494, lower limit=u8 0 ("upper limit")) -> (In Range?=w491:bool)  [unwired: 1 out]
                      n259 = Compound Arithmetic op=OR(w519, w518, w507) -> (w485:u32)
                      n260 = Compound Arithmetic op=OR(w487, w488, w489) -> (w500:bool)
                      n261 = Less?(x=w485, y=w484) -> (x < y?=w501:bool)
                      n262 = Select(t=w500, s=w501, f=TRUE) -> (s? t:f=w498:bool)
                      n263 = And(x=w498, y=w491) -> (x .and. y?=w490:bool)
                    }
                    frame #1 {
                      n264 = case shown="True" w530 {
                        tunnel: w529 -> [_ w537]
                        tunnel: w528 -> [_ w536]
                        tunnel: w527 -> [_ w535]
                        tunnel: w526 -> [_ w534]
                        tunnel: w525 -> [_ w533]
                        tunnel: w524 -> [_ w532]
                        tunnel: w523 -> [_ w531]
                        frame #0 {
                        }
                        frame #1 {
                          n265 = stacked-sequence {
                            tunnel: w537 -> [w545]
                            tunnel: w536 -> [w544]
                            tunnel: w535 -> [w543]
                            tunnel: w534 -> [w542]
                            tunnel: w533 -> [w541]
                            tunnel: w532 -> [w540]
                            tunnel: w531 -> [w538]
                            frame #0 {
                              n266 = Format Into String(format string="1. MAT: %d\n2. MAT: %d\nrouter: %d\ngap %b\noverflow %b\ninvalid %b", w545, w544, w543, w542, w541, w540) -> (resulting string=w548:string)  [unwired: 2 in, 1 out]
                              n267 = call <vilib>:"Three Button Dialog.vi"("Allow user to close window? (TRUE)"=FALSE, "message"=w548) -> ("Which Button?"=w546:T5)  [unwired: 9 in]
                              n268 = case shown="\"Left Button\", Default" w546 {
                                tunnel: w538 -> [_ w549 _]
                                tunnel: [_ w549 _] -> _
                                frame #0 {
                                }
                                frame #1 {
                                }
                                frame #2 {
                                n269 = Stop(stop? (T)=TRUE) -> ()
                                }
                              }
                            }
                          }
                        }
                      }
                    }
                  }
                }
              }
            }
          }
        }
      }
    }
    frame #2 {
      n270 = property class="VI"("Front Panel Window:Open"=FALSE) -> ()  [unwired: 2 in, 2 out]
    }
  }
